vi "RemoveDup_Rows.vi"(11 "2d Array":dbl[][](array[numeric])) -> (3 "Array With Dup Rows Removed":dbl[][](array[numeric]))   [LabVIEW 2016]
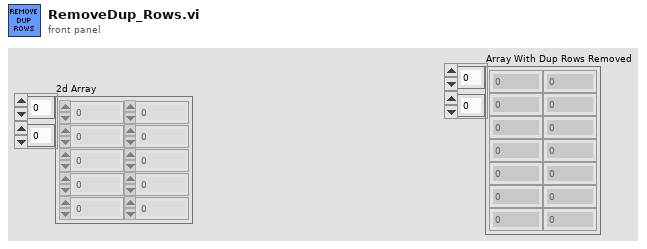
[diagram p1: front panel]
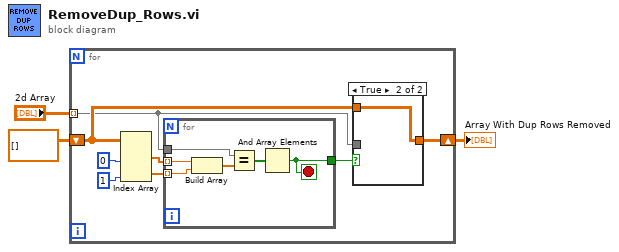
[diagram p0: block diagram]
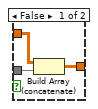
[diagram p2: hidden frame]
diagram:
  n1 = for {
    tunnel: "2d Array" -> [w5] mode=indexing
    shift-right: [w11] -> w1
    shift-left: dbl[][] [] -> [w10]
    n2 = Index Array(array=w10, index (col) #1=0 ("index"), index (col) #2=1 ("index")) -> (element #1=w7:dbl[], element #2=w6:dbl[])  [unwired: 2 in]
    n3 = for {
      tunnel: w7 -> [w20] mode=indexing
      tunnel: w6 -> [w21] mode=indexing
      tunnel: w5 -> [w18]
      tunnel: [w16] -> w4
      stop <- w16 stop-if-true
      n4 = Build Array(w20, w21) -> (w19:dbl[])
      n5 = Equal?(x=w18, y=w19) -> (x = y?=w17:bool[])
      n6 = And Array Elements(Boolean array=w17) -> (logical AND=w16:bool)
    }
    n7 = case shown="True" w4 {
      tunnel: [w14 w15] -> w11
      tunnel: w10 -> [w13 w15]
      tunnel: w5 -> [w12 _]
      frame False {
        n8 = Build Array (concatenate)(w13, w12) -> (w14:dbl[][])
      }
      frame True {
      }
    }
  }
  "Array With Dup Rows Removed" <- w1
